vi "svl_Get Terminal Name with Device Prefix.vi"(8 "error in (no error)":errorcluster, 10 "local terminal name":string, 11 "task/channels in":refnum<k21>) -> (0 "error out":errorcluster, 2 "terminal name with device prefix":tag, 3 "task out":refnum<k21>)   [LabVIEW 2017]
doc: "This example takes in a DAQmx Task and a terminal and converts this to a terminal which includes the device prefix specified in the DAQmx Physical Channel Control.\n\nFor example: \nDAQmx Task/channels in=Dev1/ai1:2\nTerminal=ai/StartTrigger\nDevice+Terminal=/Dev1/ai/StartTrigger"
uses:
  <resource>/objmgr/daqmx.rc
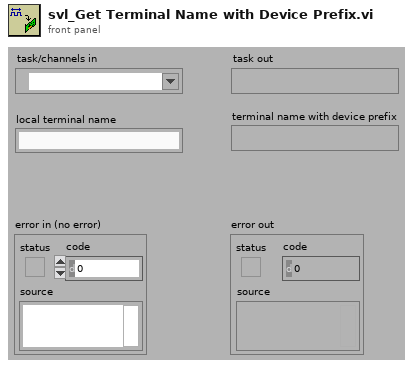
[diagram p1: front panel]
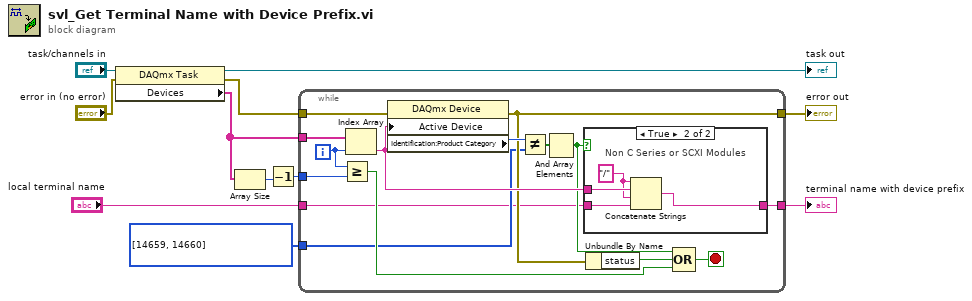
[diagram p0: block diagram]
diagram:
  w4 = i32[] [14659, 14660] items=["M Series DAQ"=14643, "E Series DAQ"=14642, "S Series DAQ"=14644, "B Series DAQ"=14662, "SC Series DAQ"=14645, "USB DAQ"=14646, "AO Series"=14647, "Digital I/O"=14648, "TIO Series"=14661, "Dynamic Signal Acquisition"=14649, "Switches"=14650, "C Series Chassis"=14658, "C Series Module"=14659, "SCXI Module"=14660, "Unknown"=12588]
  n1 = property class="DAQmx Task"(reference="task/channels in", error in="error in (no error)") -> (reference out=→"task out":refnum<k21>, error out=w3:errorcluster, "Devices"=w6:tag[])
  n2 = Array Size(array=w6) -> (size(s)=w9:i32)
  n3 = Decrement(x=w9) -> (x-1=w8:i32)
  n4 = while {
    tunnel: w6 -> [w26]
    tunnel: w3 -> [w22]
    tunnel: [w21] -> w5
    tunnel: w8 -> [w19]
    tunnel: w4 -> [w14]
    tunnel: "local terminal name" -> [w13]
    tunnel: [w12] -> w1
    i -> [w20]
    stop <- w15 stop-if-true
    n5 = Greater Or Equal?(x=w20, y=w19) -> (x >= y?=w16:bool)
    n6 = Index Array(array=w26, index=w20) -> (element=w23:tag)
    n7 = property class="DAQmx Device"(error in=w22, "Active Device"=w23) -> (error out=w21:errorcluster, "Identification:Product Category"=w25:i32)  [unwired: 1 in, 1 out]
    n8 = Not Equal?(x=w25, y=w14) -> (x != y?=w24:bool[])
    n9 = And Array Elements(Boolean array=w24) -> (logical AND=w18:bool)
    n10 = case shown="True" w18 {
      tunnel: w23 -> [_ w31]
      tunnel: w13 -> [w27 w29]
      tunnel: [w27 w28] -> w12
      frame False {
        # "Module Case do nothing"
      }
      frame True {
        w30 = "/" ("string")
        # "Non C Series or SCXI Modules"
        n11 = Concatenate Strings(w30, w31, w30, w29) -> (w28:string)
      }
    }
    n12 = Unbundle By Name(w21) -> ("status"=w17:bool)
    n13 = Compound Arithmetic op=OR(w18, w17, w16) -> (w15:bool)
  }
  "terminal name with device prefix" <- w1
  "error out" <- w5
